vi "Update Status.vi"(8 "error in (no error)":errorcluster, 10 "Status":string, 11 "Execution UI In":refnum<class "Execution UI.lvclass">) -> (0 "error out":errorcluster, 3 "Execution UI Out":refnum<class "Execution UI.lvclass">)   [LabVIEW 2020, in "Execution UI.lvclass"]
uses:
  Execution UI.lvclass
  Application Framework/Process Classes/Process/Process.lvclass
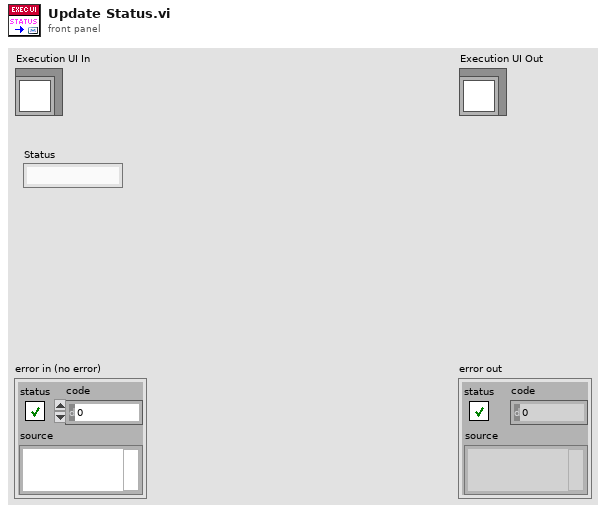
[diagram p1: front panel]
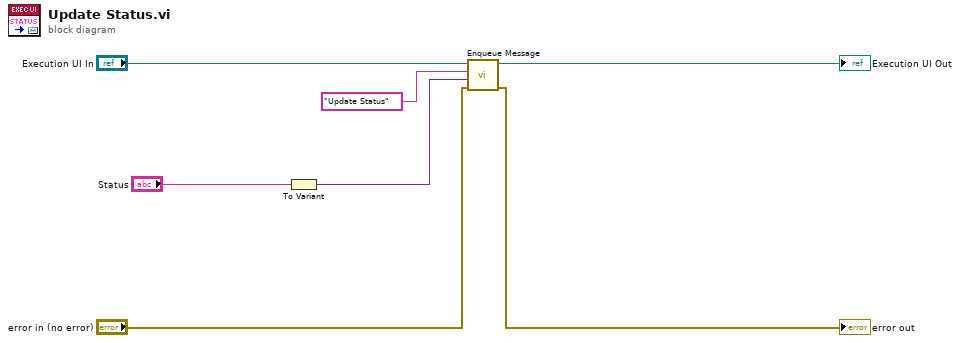
[diagram p0: block diagram]
diagram:
  n1 = To Variant(anything="Status") -> (Variant=w3:variant)
  n2 = call "Enqueue Message.vi"("error in (no error)"="error in (no error)", "Message Data"=w3, "Message"="Update Status", "Process In"="Execution UI In") -> ("error out"=→"error out":errorcluster, "Process Out"=→"Execution UI Out":refnum<class "Execution UI.lvclass">)  [unwired: 6 in]
